vi "flush comms fifos.vi"(8 "error in":errorcluster, 11 "loop comms in":T1) -> (0 "error out":errorcluster, 3 "loop comms out":T1)   [LabVIEW 2013, in "main engine.lvlib"]
uses:
  main engine.lvlib
  loop comms.ctl
  message to engine.ctl
  message request type.ctl
  message from engine.ctl
  message response type.ctl
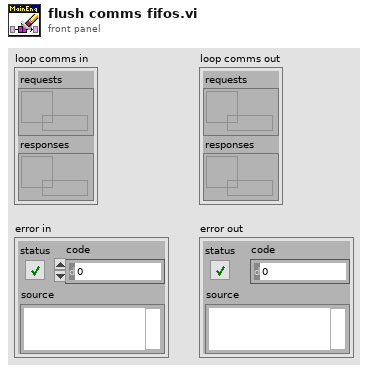
[diagram p1: front panel]
types:
  T1 = typedef "main engine.lvlib/loop comms.ctl" = cluster{"requests":refnum<k33>, "responses":refnum<k33>}
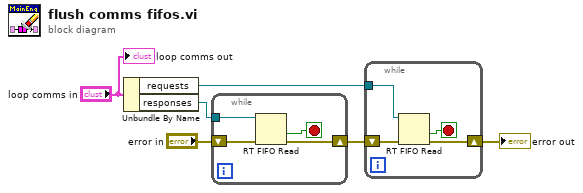
[diagram p0: block diagram]
diagram:
  n1 = Unbundle By Name("loop comms in") -> ("requests"=w2:refnum<k33>, "responses"=w5:refnum<k33>)
  n2 = while {
    tunnel: w5 -> [w10]
    shift-right: [w8] -> w3
    shift-left: "error in" -> [w9]
    stop <- w7 stop-if-true
    n3 = RT FIFO Read(0:w10, 3:w9) -> (10:w7:bool, 11:w8:errorcluster)  [unwired: 2 in, 3 out]
  }
  n4 = while {
    tunnel: w2 -> [w14]
    shift-right: [w12] -> w1
    shift-left: w3 -> [w13]
    stop <- w11 stop-if-true
    n5 = RT FIFO Read(0:w14, 3:w13) -> (10:w11:bool, 11:w12:errorcluster)  [unwired: 2 in, 3 out]
  }
  "error out" <- w1
  "loop comms out" <- "loop comms in"
